vi "Process PWM.vi"(1 "input":dbl) -> (0 "output":dbl[](array[numeric]))   [LabVIEW 2021]
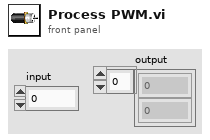
[diagram p1: front panel]
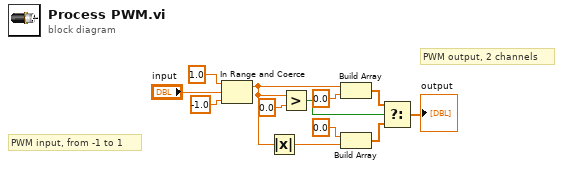
[diagram p0: block diagram]
diagram:
  # "PWM output, 2 channels"
  # "PWM input, from -1 to 1"
  n1 = In Range and Coerce(upper limit=1.0, x="input", lower limit=-1.0) -> (coerced(x)=w1:dbl)  [unwired: 1 out]
  n2 = Absolute Value(x=w1) -> (abs(x)=w2:dbl)
  n3 = Greater?(x=w1, y=0.0) -> (0:w12:bool)
  n4 = Build Array(w1, 0.0 ("element")) -> (w8:dbl[])
  n5 = Build Array(0.0 ("element"), w2) -> (w7:dbl[])
  n6 = Select(t=w8, s=w12, f=w7) -> (s? t:f=→"output":dbl[])
